vi "time_to_stop_optimization.vi"(6 "Iterations":i32, 7 "Previous Phic":dbl, 8 "Error In":errorcluster, 9 "New Thetac":dbl, 10 "Previous Thetac":dbl, 11 "New Phic":dbl) -> (0 "Error Out":errorcluster, 3 "Stop?":bool)   [LabVIEW 2019]
doc: "Determines if it is time to stop optimization of the c-axis. Both varaibles must change by less that or equal to 0.005. Also stops if we reach 2000 iterations of optimization."
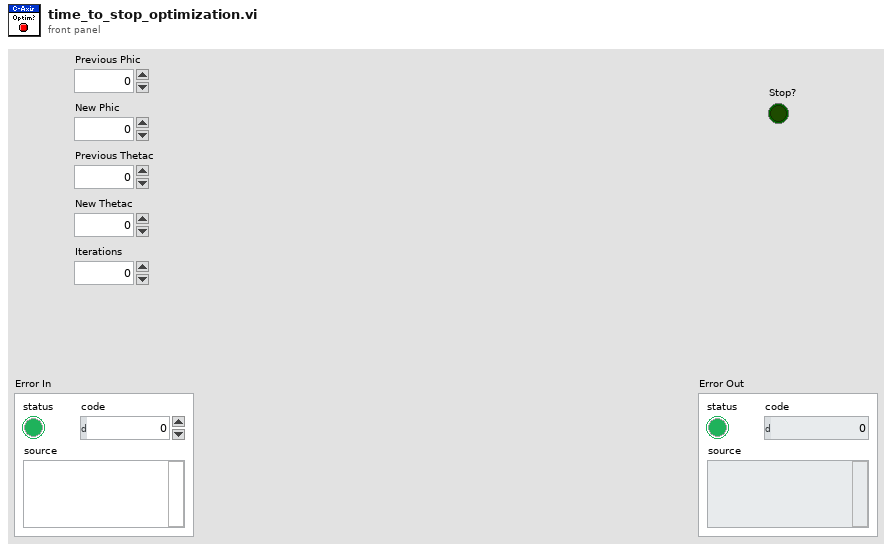
[diagram p1: front panel]
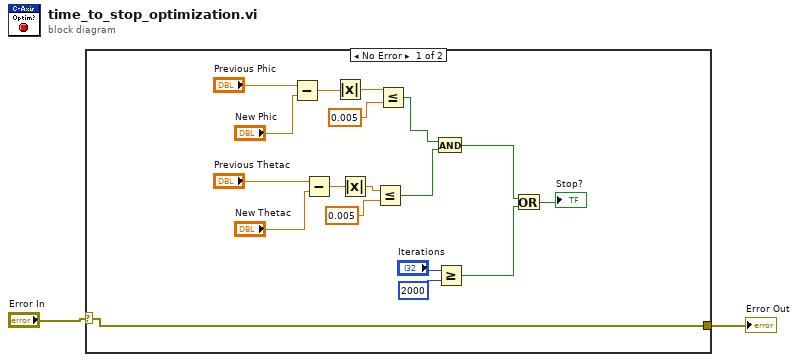
[diagram p0: block diagram]
diagram:
  n1 = case shown="No Error" "Error In" {
    selector: "Error In" -> [w3 w21]
    tunnel: [w3 w21] -> w1
    frame No Error {
      n2 = Subtract(x="Previous Phic", y="New Phic") -> (x-y=w13:dbl)
      n3 = Subtract(x="Previous Thetac", y="New Thetac") -> (x-y=w12:dbl)
      n4 = Absolute Value(x=w13) -> (abs(x)=w11:dbl)
      n5 = Absolute Value(x=w12) -> (abs(x)=w8:dbl)
      n6 = Less Or Equal?(x=w8, y=0.005) -> (x <= y?=w6:bool)
      n7 = Less Or Equal?(x=w11, y=0.005) -> (x <= y?=w7:bool)
      n8 = And(x=w7, y=w6) -> (x .and. y?=w5:bool)
      n9 = Greater Or Equal?(x="Iterations", y=2000) -> (x >= y?=w4:bool)
      n10 = Or(x=w5, y=w4) -> (x .or. y?=→"Stop?":bool)
    }
    frame Error {
    }
  }
  "Error Out" <- w1
